vi "TcA01-006_ObjectsCanBeNamedWhenCreated.vi"(1 "Input buffer":T3="1", 3 "Invocation info":T2, 5 "error in (no error)":errorcluster, 6 "Add log to result?":bool) -> (16 "Test Data":T1 {"Numeric Measurement" format="%.2f"}, 19 "error out":errorcluster)   [LabVIEW 2020]
doc: "Test case template."
uses:
  Shared/Support_InputBuffer.ctl
  Shared/Support_InvocationInfo.ctl
  Shared/Support_TestData.ctl
  <vilib>/addons/_AddQ/G#Object/utils/G#Object_CreateMethod.ctl
  TestClasses/G#BaseClass1_class/G#BaseClass1.lvclass
  TestClasses/G#SubClass1_class/G#SubClass1.lvclass
  <vilib>/addons/_AddQ/G#Object/G#Object.lvclass
panel:
  in  "Test name":string="TcA01-006 Objects can be named when created"
  out "Test result":bool
  out "Result":string
  # "Verify that objects within a class can be named when created\nand that there can only exist one object by that name within a class."
  # "Sub test case"
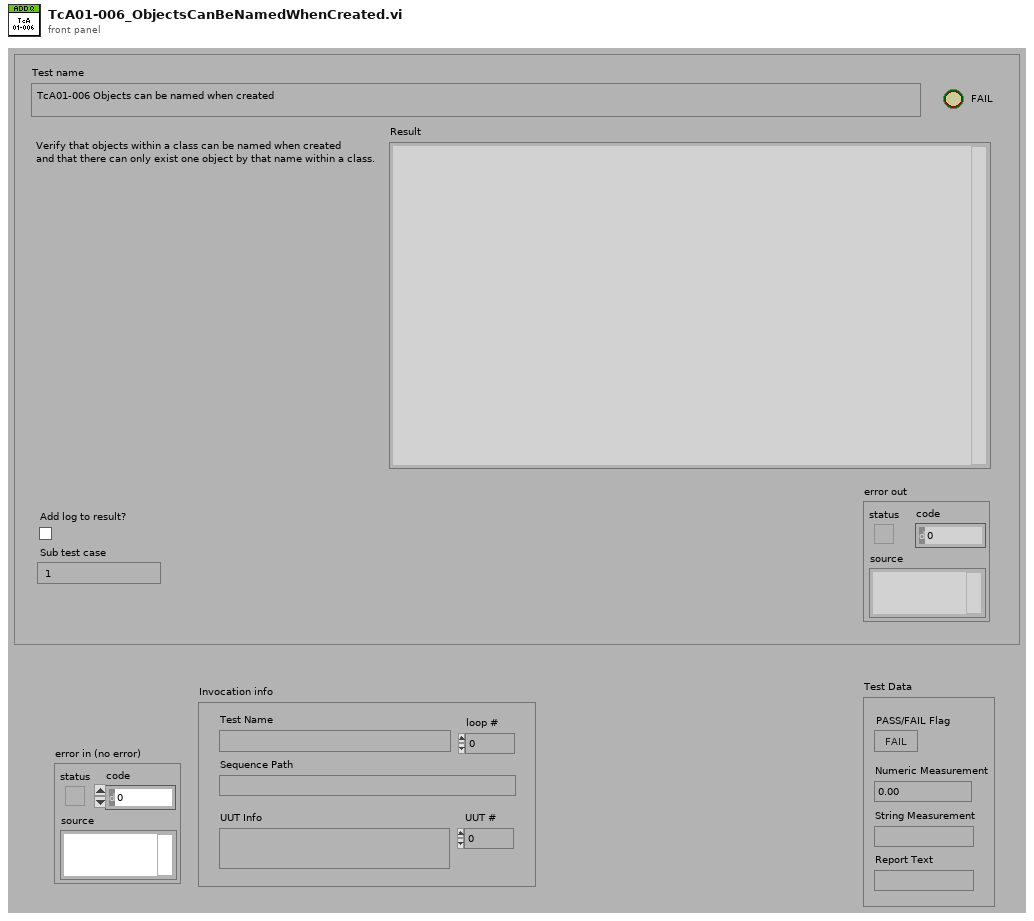
[diagram p1: front panel]
types:
  T1 = typedef "Support_TestData.ctl" = cluster{"PASS/FAIL Flag":bool, "Numeric Measurement":dbl, "String Measurement":string, "Report Text":string}
  T2 = typedef "Support_InvocationInfo.ctl" = cluster{"UUT #":i32, "loop #":i32, "UUT Info":string, "Test Name":string, "Sequence Path":path}
  T3 = typedef "Support_InputBuffer.ctl" = string
  T4 = typedef "G#Object.lvclass/G#Object_CreateMethod.ctl" = enum16{"Create", "Create or look up existing", "Look up existing"}
  T5 = typedef "Support_ResultType.ctl" = cluster{"Pass":bool, "Comment":string, "MeasurementValue":dbl}
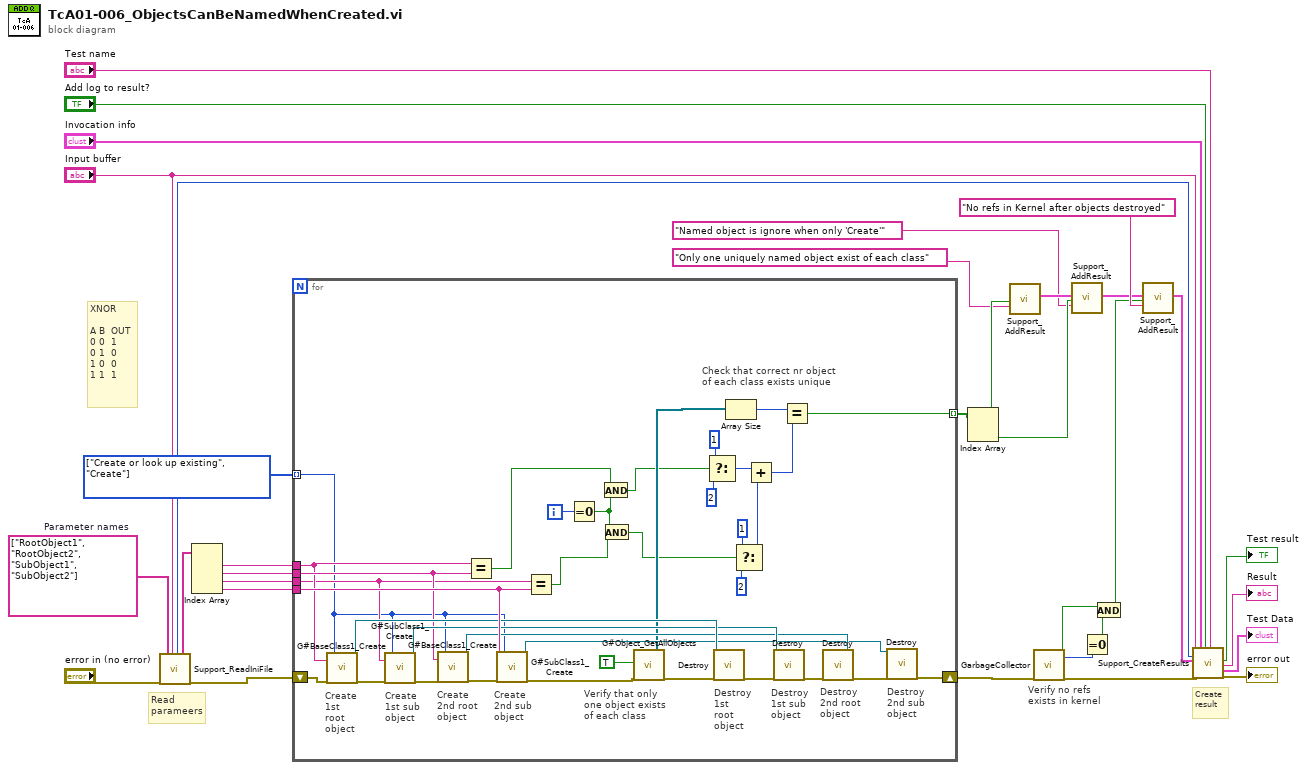
[diagram p0: block diagram]
diagram:
  w8 = T4[] [enum."Create or look up existing", enum."Create"] items=["Create", "Create or look up existing", "Look up existing"]
  w25 = string[] ["RootObject1", "RootObject2", "SubObject1", "SubObject2"]  # Parameter names
  # "XNOR\n\nA B  OUT\n0 0  1\n0 1  0\n1 0  0\n1 1  1"
  # "Verify no refs\nexists in kernel"
  # "Read\nparameers"
  # "Create\nresult"
  n1 = call "Support_ReadIniFile.vi"("error in (no error)"="error in (no error)", "Parameter names"=w25, "Sub test case"="Input buffer") -> ("Timer start"=w23:u32, "Parameters as string"=w21:string[], "error out"=w22:errorcluster)  [unwired: 9 in, 5 out]
  n2 = Index Array(array=w21) -> (element #1=w15:string, element #2=w16:string, element #3=w14:string, element #4=w19:string)  [unwired: 4 in]
  n3 = for {
    tunnel: w19 -> [w67]
    tunnel: w16 -> [w62]
    tunnel: w15 -> [w61]
    tunnel: w14 -> [w60]
    tunnel: w8 -> [w47] mode=indexing
    shift-right: [w41] -> w9
    shift-left: w22 -> [w69]
    tunnel: [w34] -> w5 mode=indexing
    i -> [w40]
    # "Check that correct nr object\nof each class exists unique"
    # "Verify that only\none object exists\nof each class"
    # "Create\n1st root\nobject"
    # "Create\n2nd root\nobject"
    # "Create\n1st sub \nobject"
    # "Create\n2nd sub\nobject"
    # "Destroy\n2nd sub\nobject"
    # "Destroy\n1st sub \nobject"
    # "Destroy\n2nd root\nobject"
    # "Destroy\n1st root\nobject"
    n4 = call "G#BaseClass1_Create.vi"("object name"=w61, "error in (no error)"=w69, "create method"=w47) -> ("reference out"=w66:refnum<class "G#BaseClass1.lvclass">, "error out"=w46:errorcluster)  [unwired: 14 in, 1 out]
    n5 = call "G#SubClass1_Create.vi"("object name"=w60, "error in (no error)"=w46, "create method"=w47) -> ("reference out"=w65:refnum<class "G#SubClass1.lvclass">, "error out"=w45:errorcluster)  [unwired: 14 in, 1 out]
    n6 = call "G#BaseClass1_Create.vi"("object name"=w62, "error in (no error)"=w45, "create method"=w47) -> ("reference out"=w64:refnum<class "G#BaseClass1.lvclass">, "error out"=w44:errorcluster)  [unwired: 14 in, 1 out]
    n7 = Equal?(x=w61, y=w62) -> (x = y?=w39:bool)
    n8 = call "G#SubClass1_Create.vi"("object name"=w67, "error in (no error)"=w44, "create method"=w47) -> ("reference out"=w63:refnum<class "G#SubClass1.lvclass">, "error out"=w43:errorcluster)  [unwired: 14 in, 1 out]
    n9 = Equal?(x=w60, y=w67) -> (x = y?=w36:bool)
    n10 = Equal To 0?(x=w40) -> (x = 0?=w37:bool)
    n11 = And(x=w39, y=w37) -> (x .and. y?=w38:bool)
    n12 = And(x=w37, y=w36) -> (x .and. y?=w35:bool)
    n13 = call <vilib>:"G#Object_GetAllObjects.vi"("only refs (F)"=TRUE ("only refs"), "error in (no error)"=w43) -> ("all refs"=w49:refnum<class "G#Object.lvclass">[], "error out"=w50:errorcluster)  [unwired: 14 in, 2 out]
    n14 = Select(t=1 ("f"), s=w38, f=2) -> (s? t:f=w53:i32)
    n15 = call-dynamic "Destroy.vi"("reference in"=w66, "error in (no error)"=w50) -> ("error out"=w59:errorcluster)  [unwired: 16 in, 1 out]
    n16 = Array Size(array=w49) -> (size(s)=w68:i32)
    n17 = Select(t=1 ("f"), s=w35, f=2) -> (s? t:f=w52:i32)
    n18 = Add(x=w53, y=w52) -> (x+y=w51:i32)
    n19 = call-dynamic "Destroy.vi"("reference in"=w65, "error in (no error)"=w59) -> ("error out"=w58:errorcluster)  [unwired: 16 in, 1 out]
    n20 = Equal?(x=w68, y=w51) -> (x = y?=w34:bool)
    n21 = call-dynamic "Destroy.vi"("reference in"=w64, "error in (no error)"=w58) -> ("error out"=w42:errorcluster)  [unwired: 16 in, 1 out]
    n22 = call-dynamic "Destroy.vi"("reference in"=w63, "error in (no error)"=w42) -> ("error out"=w41:errorcluster)  [unwired: 16 in, 1 out]
  }
  n23 = Index Array(array=w5) -> (element #1=w4:bool, element #2=w3:bool)  [unwired: 2 in]
  n24 = call "Support_AddResult.vi"("Pass"=w4, "Comment"="Only one uniquely named object exist of each class") -> ("Results out"=w6:T5[])  [unwired: 17 in]
  n25 = call <vilib>:"GarbageCollector.vi"("error in (no error)"=w9) -> ("OK"=w11:bool, "# of objects killed"=w13:i32, "error out"=w17:errorcluster)  [unwired: 16 in]
  n26 = call "Support_AddResult.vi"("Results in"=w6, "Pass"=w3, "Comment"="Named object is ignore when only 'Create'") -> ("Results out"=w7:T5[])  [unwired: 16 in]
  n27 = Equal To 0?(x=w13) -> (x = 0?=w12:bool)
  n28 = And(x=w11, y=w12) -> (x .and. y?=w10:bool)
  n29 = call "Support_AddResult.vi"("Results in"=w7, "Pass"=w10, "Comment"="No refs in Kernel after objects destroyed") -> ("Results out"=w20:T5[])  [unwired: 16 in]
  n30 = call "Support_CreateResults.vi"("Sub test case"="Input buffer", "Timer start"=w23, "Results"=w20, "error in (no error)"=w17, "Invocation info"="Invocation info", "Add log to result?"="Add log to result?", "Test name"="Test name") -> ("Pass/fail flag"=→"Test result":bool, "Result"=→"Result":string, "Test Data"=→"Test Data":T1, "error out"=→"error out":errorcluster)  [unwired: 9 in]
